vi "Finalize.vi"(8 "error in (no error)":errorcluster, 11 "Loopback in":refnum<class "Loopback.lvclass">) -> (0 "error out":errorcluster, 3 "Loopback out":refnum<class "Loopback.lvclass">)   [LabVIEW 2020, in "Loopback.lvclass"]
uses:
  Loopback.lvclass
  Loopback.lvclass/Loopback.ctl
  <vilib>/FPGAPlugInAG/Dynamic/niLvFpga_Close_Dynamic.vi
  <vilib>/rvi/interface/nirviCloseFPGA/nirviCloseFPGA.xnode
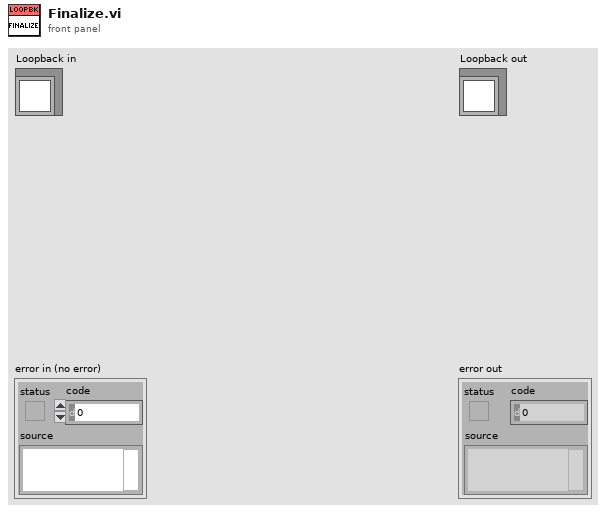
[diagram p1: front panel]
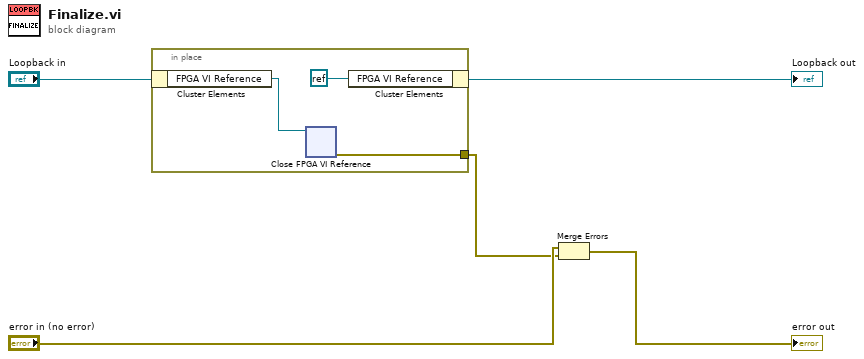
[diagram p0: block diagram]
diagram:
  n1 = in-place {
    in-place-border: [w8] -> w1
    n2 = in-place-cluster #1("Loopback in") -> ("FPGA VI Reference"=w7:refnum<k20>)
    n3 = xnode "Close FPGA VI Reference"("FPGA VI Reference In"=w7) -> ("error out"=w8:errorcluster)  [unwired: 1 in]
    n4 = in-place-cluster #1("FPGA VI Reference"=refnum<k0> refnum) -> (→"Loopback out":refnum<class "Loopback.lvclass">)
  }
  n5 = Merge Errors("error in (no error)", w1) -> (→"error out":errorcluster)
